vi "Main.vi"() -> ()   [LabVIEW 2018] (continued)
                w3602 = u8 132 items=["I/O (P)"=128, "Input (I)"=129, "Output (Q)"=130, "Bit Memory (M)"=131, "Data (DB)"=132, "Instance Data (DI)"=133, "Local Data (L)"=134, "Predecessor Local Data (VL)"=135] ("寄存器类型")
                w3601 = u16 1 items=["byte", "word", "Dword"] ("数据类型")
                n980 = Index Array(array=w3596) -> (element=w3595:string)  [unwired: 1 in]
                n981 = Decimal String To Number(string=w3595, default (0L)=u32 0 ("默认(0 I32)")) -> (number=w3605:u32)  [unwired: 1 in, 1 out]
                n982 = call "S7_Write.vi"("TCP"=w3597, "寄存器类型"=w3602, "DB #"=u16 20, "写入地址"=u32 2, "数据类型"=w3601, "写入数据"=w3605) -> ("TCP"=w3599:refnum<k5>, "error out"=w3598:errorcluster)  [unwired: 7 in, 1 out]
              }
            }
            "扫码请求回复401" <- w3555
            n983 = Bundle By Name(cluster=w3554, "扫码超时1"=w3555) -> (w3553:T7)
          }
          frame "-------------" {
          }
          frame "读数据保存请求" {
            w3639 = u16 0 items=["byte", "word", "Dword"] ("数据类型")
            w3641 = u8 132 items=["I/O (P)"=128, "Input (I)"=129, "Output (Q)"=130, "Bit Memory (M)"=131, "Data (DB)"=132, "Instance Data (DI)"=133, "Local Data (L)"=134, "Predecessor Local Data (VL)"=135] ("寄存器类型")
            n984 = call "S7_Read.vi"("TCP"=w3631, "DB #"=u16 20, "读取长度"=u16 1, "寄存器类型"=w3641, "起始地址"=u32 0, "数据类型"=w3639) -> ("TCP"=w3630:refnum<k5>, "数据"=w3636:u32[], "error out"=w3629:errorcluster)  [unwired: 6 in, 1 out]
            n985 = Index Array(array=w3636, index=0 ("索引")) -> (element=w3634:u32)
            n986 = Number To Boolean Array(number=w3634) -> (Boolean array=w3633:bool[])
            n987 = Unbundle By Name(w3612) -> ("数据保存超时1"=w3613:string)
            n988 = Index Array(array=w3633, index=1 ("索引")) -> (element=w3618:bool)
            "ST401数据读取" <- w3618
            n989 = Not Equal?(x=w3613, y="999") -> (x != y?=w3615:bool)
            n990 = Not(x=w3615) -> (.not. x?=w3616:bool)
            n991 = call <vilib>:"Boolean Crossing PtByPt.vi"("direction"=enum16{"either", "false-true", "true-false"}."false-true", "input"=w3618) -> ("crossing"=w3622:bool)  [unwired: 1 in]
            n992 = call <vilib>:"Boolean Crossing PtByPt.vi"("direction"=enum16{"either", "false-true", "true-false"}."true-false", "input"=w3618) -> ("crossing"=w3623:bool)  [unwired: 1 in]
            n993 = call "已用时间10"("Reset"=w3616) -> ("Time has Elapsed"=w3617:bool)  [unwired: 11 in, 7 out]
            n994 = Insert Into Array(array=bool[] [] ("数组"), index=0 ("索引"), new element #1=w3622, new element #2=w3623) -> (w3626:bool[])
            n995 = Boolean Array To Number(Boolean array=w3626) -> (number=w3627:u32)
            n996 = case shown="2" w3627 {
              tunnel: [cluster{"Data":string[], "State":T1} {"Data"=[], "State"=enum."读扫码请求3"} ("元素") w3646 w3650] -> w3619
              tunnel: w3611 -> [_ w3647 w3651]
              frame 0, Default {
              }
              frame 1 {
                w3646 = cluster{"Data":string[], "State":T1} {"Data"=[], "State"=enum."读数据"} ("元素")
                n997 = Enqueue Element(queue=w3647, element=w3646, timeout in ms (-1)=10 ("超时毫秒(-1)")) -> ()  [unwired: 1 in, 3 out]
              }
              frame 2 {
                w3650 = cluster{"Data":string[], "State":T1} {"Data"=["999"], "State"=enum."数据保存回复"} ("元素")
                n998 = Enqueue Element(queue=w3651, element=w3650, timeout in ms (-1)=10 ("超时毫秒(-1)")) -> ()  [unwired: 1 in, 3 out]
              }
            }
            n999 = case shown="真" w3617 {
              tunnel: w3611 -> [_ w3643]
              frame False {
              }
              frame True {
                n1000 = Enqueue Element(queue=w3643, element=cluster{"Data":string[], "State":T1} {"Data"=["999"], "State"=enum."数据保存回复"} ("元素"), timeout in ms (-1)=10 ("超时毫秒(-1)")) -> ()  [unwired: 1 in, 3 out]
              }
            }
          }
          frame "读数据" {
            w3657 = u16 0 items=["byte", "word", "Dword"] ("数据类型")
            w3659 = u8 132 items=["I/O (P)"=128, "Input (I)"=129, "Output (Q)"=130, "Bit Memory (M)"=131, "Data (DB)"=132, "Instance Data (DI)"=133, "Local Data (L)"=134, "Predecessor Local Data (VL)"=135] ("寄存器类型")
            w3694 = u16 1 items=["byte", "word", "Dword"] ("数据类型")
            w3690 = u8 132 items=["I/O (P)"=128, "Input (I)"=129, "Output (Q)"=130, "Bit Memory (M)"=131, "Data (DB)"=132, "Instance Data (DI)"=133, "Local Data (L)"=134, "Predecessor Local Data (VL)"=135] ("寄存器类型")
            n1001 = call "S7_Read.vi"("TCP"=w3656, "DB #"=u16 20, "读取长度"=u16 1, "寄存器类型"=w3659, "起始地址"=u32 0, "数据类型"=w3657) -> ("TCP"=w3655:refnum<k5>, "数据"=w3666:u32[], "error out"=w3654:errorcluster)  [unwired: 6 in, 1 out]
            n1002 = Index Array(array=w3666, index=0 ("索引")) -> (element=w3667:u32)
            n1003 = Number To Boolean Array(number=w3667) -> (Boolean array=w3668:bool[])
            n1004 = Index Array(array=w3668, index=7 ("索引")) -> (element=w3665:bool)
            n1005 = Equal?(x=w3665, y=TRUE) -> (x = y?=w3653:bool)
            n1006 = case shown="真" w3653 {
              tunnel: [" " "Y"] -> w3652
              frame False {
              }
              frame True {
              }
            }
            n1007 = call "S7_Read.vi"("TCP"=w3655, "DB #"=u16 20, "读取长度"=u16 1, "寄存器类型"=w3690, "起始地址"=u32 6, "数据类型"=w3694, "error in"=w3654) -> ("TCP"=w3676:refnum<k5>, "数据"=w3689:u32[], "error out"=w3679:errorcluster)  [unwired: 5 in, 1 out]
            n1008 = Index Array(array=w3689) -> (element=w3678:u32)  [unwired: 1 in]
            n1009 = Equal?(x=w3678, y=u32 1) -> (x = y?=w3687:bool)
            n1010 = case shown="假" w3687 {
              tunnel: ["NG" "OK"] -> w3677
              frame False {
              }
              frame True {
              }
            }
            n1011 = Format Date/Time String(time format string (%c)="%Y-%m-%d" ("时间格式字符串(%c)")) -> (date/time string=w3681:string)  [unwired: 2 in]
            n1012 = Get Date/Time String() -> (time string=w3680:string)  [unwired: 3 in, 1 out]
            n1013 = Insert Into Array(array=string[] [] ("数组"), index=0 ("索引"), new element #1="401" ("新元素/子数组"), new element #2=w3677, new element #3=w3681, new element #4=w3680, new element #5=w3677, new element #6=w3652) -> (w3686:string[])
            n1014 = Enqueue Element(queue=w3675, element=w3686, error in (no error)=w3679) -> (error out=w3671:errorcluster)  [unwired: 1 in, 2 out]
            n1015 = property on="ST401数据读取（事件）" class="Bool (严格)"(error in=w3671, "Val(Sgnl)"=TRUE ("值(信号)")) -> (error out=w3670:errorcluster)  [unwired: 1 in, 1 out]
          }
          frame "数据保存回复" {
            w3712 = u8 132 items=["I/O (P)"=128, "Input (I)"=129, "Output (Q)"=130, "Bit Memory (M)"=131, "Data (DB)"=132, "Instance Data (DI)"=133, "Local Data (L)"=134, "Predecessor Local Data (VL)"=135] ("寄存器类型")
            w3713 = u16 1 items=["byte", "word", "Dword"] ("数据类型")
            n1016 = Index Array(array=w3706, index=0 ("索引")) -> (element=w3699:string)
            "数据保存请求回复401" <- w3699
            n1017 = Decimal String To Number(string=w3699, default (0L)=u32 0 ("默认(0 I32)")) -> (number=w3708:u32)  [unwired: 1 in, 1 out]
            n1018 = call "S7_Write.vi"("TCP"=w3707, "寄存器类型"=w3712, "DB #"=u16 20, "写入地址"=u32 4, "数据类型"=w3713, "写入数据"=w3708) -> ("TCP"=w3704:refnum<k5>, "error out"=w3705:errorcluster)  [unwired: 7 in, 1 out]
            n1019 = Bundle By Name(cluster=w3701, "数据保存超时1"=w3699) -> (w3700:T7)
          }
          frame "-----------------" {
          }
          frame "错误" {
            n1020 = Flush Queue(queue=w3722) -> ()  [unwired: 1 in, 3 out]
            n1021 = Flush Queue(queue=w3721) -> ()  [unwired: 1 in, 3 out]
            n1022 = call "S7_Close.vi"("TCP Connection Ref"=w3725) -> ("error out"=w3723:errorcluster)  [unwired: 10 in]
            n1023 = call <vilib>:"Clear Errors.vi"("error in (no error)"=w3723) -> ()  [unwired: 5 in, 2 out]
          }
          frame "退出" {
            n1024 = Release Queue(queue=w3734) -> ()  [unwired: 2 in, 3 out]
            n1025 = Release Queue(queue=w3733) -> ()  [unwired: 2 in, 3 out]
            n1026 = call "S7_Close.vi"("TCP Connection Ref"=w3732) -> ("error out"=w3731:errorcluster)  [unwired: 10 in]
          }
          frame "-------------------" {
          }
          frame "读扫码请求2" {
            w3770 = u16 0 items=["byte", "word", "Dword"] ("数据类型")
            w3772 = u8 132 items=["I/O (P)"=128, "Input (I)"=129, "Output (Q)"=130, "Bit Memory (M)"=131, "Data (DB)"=132, "Instance Data (DI)"=133, "Local Data (L)"=134, "Predecessor Local Data (VL)"=135] ("寄存器类型")
            n1027 = call "S7_Read.vi"("TCP"=w3753, "DB #"=u16 20, "读取长度"=u16 1, "寄存器类型"=w3772, "起始地址"=u32 0, "数据类型"=w3770) -> ("TCP"=w3752:refnum<k5>, "数据"=w3767:u32[], "error out"=w3751:errorcluster)  [unwired: 6 in, 1 out]
            n1028 = Index Array(array=w3767, index=0 ("索引")) -> (element=w3765:u32)
            n1029 = Number To Boolean Array(number=w3765) -> (Boolean array=w3764:bool[])
            n1030 = Index Array(array=w3764, index=2 ("索引")) -> (element=w3754:bool)
            "ST402扫码请求" <- w3754
            n1031 = Unbundle By Name(w3743) -> ("扫码超时2"=w3744:string)
            n1032 = Not Equal?(x=w3744, y="999") -> (x != y?=w3746:bool)
            n1033 = Not(x=w3746) -> (.not. x?=w3747:bool)
            n1034 = call <vilib>:"Boolean Crossing PtByPt.vi"("direction"=enum16{"either", "false-true", "true-false"}."false-true", "input"=w3754) -> ("crossing"=w3760:bool)  [unwired: 1 in]
            n1035 = call <vilib>:"Boolean Crossing PtByPt.vi"("direction"=enum16{"either", "false-true", "true-false"}."true-false", "input"=w3754) -> ("crossing"=w3759:bool)  [unwired: 1 in]
            n1036 = call "已用时间25"("Reset"=w3747) -> ("Time has Elapsed"=w3748:bool)  [unwired: 11 in, 7 out]
            n1037 = Insert Into Array(array=bool[] [] ("数组"), index=0 ("索引"), new element #1=w3760, new element #2=w3759) -> (w3756:bool[])
            n1038 = Boolean Array To Number(Boolean array=w3756) -> (number=w3755:u32)
            n1039 = case shown="0, 默认" w3755 {
              tunnel: [cluster{"Data":string[], "State":T1} {"Data"=[], "State"=enum."读数据保存请求2"} ("元素") w3778 w3780] -> w3750
              tunnel: w3742 -> [_ w3779 w3781]
              frame 0, Default {
              }
              frame 1 {
                w3778 = cluster{"Data":string[], "State":T1} {"Data"=[], "State"=enum."读二维码2"} ("元素")
                n1040 = Enqueue Element(queue=w3779, element=w3778, timeout in ms (-1)=10 ("超时毫秒(-1)")) -> ()  [unwired: 1 in, 3 out]
              }
              frame 2 {
                w3780 = cluster{"Data":string[], "State":T1} {"Data"=["999"], "State"=enum."扫码回复2"} ("元素")
                n1041 = Enqueue Element(queue=w3781, element=w3780, timeout in ms (-1)=10 ("超时毫秒(-1)")) -> ()  [unwired: 1 in, 3 out]
              }
            }
            n1042 = case shown="真" w3748 {
              tunnel: w3742 -> [_ w3774]
              frame False {
              }
              frame True {
                n1043 = Enqueue Element(queue=w3774, element=cluster{"Data":string[], "State":T1} {"Data"=["999"], "State"=enum."扫码回复2"} ("元素"), timeout in ms (-1)=10 ("超时毫秒(-1)")) -> ()  [unwired: 1 in, 3 out]
              }
            }
          }
          frame "读二维码2" {
            n1044 = disable-structure shown="禁用" {
              disable-tunnel: w3791 -> [w3798 _]
              disable-tunnel: w3790 -> [w3797 _]
              disable-tunnel: [w3796 _] -> w3789
              disable-tunnel: [w3795 _] -> w3785
              frame Disabled {
                w3807 = u16 0 items=["byte", "word", "Dword"] ("数据类型")
                w3803 = u8 132 items=["I/O (P)"=128, "Input (I)"=129, "Output (Q)"=130, "Bit Memory (M)"=131, "Data (DB)"=132, "Instance Data (DI)"=133, "Local Data (L)"=134, "Predecessor Local Data (VL)"=135] ("寄存器类型")
                n1045 = call "S7_Read.vi"("TCP"=w3797, "DB #"=u16 20, "读取长度"=u16 17, "寄存器类型"=w3803, "起始地址"=u32 42, "数据类型"=w3807) -> ("TCP"=w3796:refnum<k5>, "数据"=w3808:u32[], "error out"=w3810:errorcluster)  [unwired: 6 in, 1 out]
                n1046 = To Unsigned Word Integer(number=w3808) -> (unsigned 16bit integer=w3809:u16[])
                n1047 = call "还原为字符串.vi"("error in (no error)"=w3810, "输入数组"=w3809) -> ("error out"=w3799:errorcluster, "字符串"=w3793:string)  [unwired: 8 in]
                n1048 = Match Pattern(string=w3793, regular expression=" " ("正则表达式")) -> (before substring=w3792:string)  [unwired: 1 in, 3 out]
                "402二维码 2" <- w3792
                n1049 = Insert Into Array(array=string[] [] ("数组"), index=0 ("索引"), new element=w3792) -> (w3800:string[])
                n1050 = Enqueue Element(queue=w3798, element=w3800, error in (no error)=w3799) -> (error out=w3795:errorcluster)  [unwired: 1 in, 2 out]
              }
              frame Enabled {
              }
            }
            n1051 = property on="ST402扫码请求(事件)" class="Bool (严格)"(error in=w3785, "Val(Sgnl)"=TRUE ("值(信号)")) -> (error out=w3784:errorcluster)  [unwired: 1 in, 1 out]
          }
          frame "扫码回复2" {
            n1052 = Array Size(array=w3819) -> (size(s)=w3820:i32)
            n1053 = case shown="3, 默认" w3820 {
              tunnel: w3819 -> [w3845 w3854]
              tunnel: w3818 -> [w3832 w3855]
              tunnel: [w3823 w3857] -> w3817
              tunnel: [w3822 w3856] -> w3816
              tunnel: [w3821 w3853] -> w3811
              frame 3, Default {
                w3835 = u8 132 items=["I/O (P)"=128, "Input (I)"=129, "Output (Q)"=130, "Bit Memory (M)"=131, "Data (DB)"=132, "Instance Data (DI)"=133, "Local Data (L)"=134, "Predecessor Local Data (VL)"=135] ("寄存器类型")
                w3834 = u16 1 items=["byte", "word", "Dword"] ("数据类型")
                w3842 = u8 132 items=["I/O (P)"=128, "Input (I)"=129, "Output (Q)"=130, "Bit Memory (M)"=131, "Data (DB)"=132, "Instance Data (DI)"=133, "Local Data (L)"=134, "Predecessor Local Data (VL)"=135] ("寄存器类型")
                w3843 = u16 1 items=["byte", "word", "Dword"] ("数据类型")
                w3849 = u8 132 items=["I/O (P)"=128, "Input (I)"=129, "Output (Q)"=130, "Bit Memory (M)"=131, "Data (DB)"=132, "Instance Data (DI)"=133, "Local Data (L)"=134, "Predecessor Local Data (VL)"=135] ("寄存器类型")
                w3848 = u16 1 items=["byte", "word", "Dword"] ("数据类型")
                n1054 = Index Array(array=w3845) -> (element #1=w3821:string, element #2=w3828:string, element #3=w3827:string)  [unwired: 3 in]
                n1055 = Equal?(x=w3827, y="OK") -> (x = y?=w3825:bool)
                n1056 = Decimal String To Number(string=w3828, default (0L)=u32 0 ("默认(0 I32)")) -> (number=w3829:u32)  [unwired: 1 in, 1 out]
                n1057 = case shown="假" w3825 {
                  tunnel: [u32 2 ("写入数据") u32 1 ("写入数据")] -> w3824
                  frame False {
                  }
                  frame True {
                  }
                }
                n1058 = call "S7_Write.vi"("TCP"=w3832, "寄存器类型"=w3849, "DB #"=u16 20, "写入地址"=u32 18, "数据类型"=w3848, "写入数据"=w3829) -> ("TCP"=w3839:refnum<k5>, "error out"=w3840:errorcluster)  [unwired: 7 in, 1 out]
                n1059 = call "S7_Write.vi"("TCP"=w3839, "寄存器类型"=w3842, "DB #"=u16 20, "写入地址"=u32 20, "数据类型"=w3843, "写入数据"=w3824, "error in"=w3840) -> ("TCP"=w3831:refnum<k5>, "error out"=w3830:errorcluster)  [unwired: 6 in, 1 out]
                n1060 = Decimal String To Number(string=w3821, default (0L)=u32 0 ("默认(0 I32)")) -> (number=w3838:u32)  [unwired: 1 in, 1 out]
                n1061 = call "S7_Write.vi"("TCP"=w3831, "寄存器类型"=w3835, "DB #"=u16 20, "写入地址"=u32 14, "数据类型"=w3834, "写入数据"=w3838, "error in"=w3830) -> ("TCP"=w3823:refnum<k5>, "error out"=w3822:errorcluster)  [unwired: 6 in, 1 out]
              }
              frame 1 {
                w3860 = u8 132 items=["I/O (P)"=128, "Input (I)"=129, "Output (Q)"=130, "Bit Memory (M)"=131, "Data (DB)"=132, "Instance Data (DI)"=133, "Local Data (L)"=134, "Predecessor Local Data (VL)"=135] ("寄存器类型")
                w3859 = u16 1 items=["byte", "word", "Dword"] ("数据类型")
                n1062 = Index Array(array=w3854) -> (element=w3853:string)  [unwired: 1 in]
                n1063 = Decimal String To Number(string=w3853, default (0L)=u32 0 ("默认(0 I32)")) -> (number=w3863:u32)  [unwired: 1 in, 1 out]
                n1064 = call "S7_Write.vi"("TCP"=w3855, "寄存器类型"=w3860, "DB #"=u16 20, "写入地址"=u32 14, "数据类型"=w3859, "写入数据"=w3863) -> ("TCP"=w3857:refnum<k5>, "error out"=w3856:errorcluster)  [unwired: 7 in, 1 out]
              }
            }
            "扫码请求回复402" <- w3811
            n1065 = Bundle By Name(cluster=w3813, "扫码超时2"=w3811) -> (w3812:T7)
          }
          frame "-- --------------" {
          }
          frame "读数据保存请求2" {
            w3882 = u8 132 items=["I/O (P)"=128, "Input (I)"=129, "Output (Q)"=130, "Bit Memory (M)"=131, "Data (DB)"=132, "Instance Data (DI)"=133, "Local Data (L)"=134, "Predecessor Local Data (VL)"=135] ("寄存器类型")
            w3881 = u16 1 items=["byte", "word", "Dword"] ("数据类型")
            w3910 = u16 0 items=["byte", "word", "Dword"] ("数据类型")
            w3912 = u8 132 items=["I/O (P)"=128, "Input (I)"=129, "Output (Q)"=130, "Bit Memory (M)"=131, "Data (DB)"=132, "Instance Data (DI)"=133, "Local Data (L)"=134, "Predecessor Local Data (VL)"=135] ("寄存器类型")
            n1066 = Unbundle By Name(w3871) -> ("看门狗"=w3879:string)
            n1067 = Decimal String To Number(string=w3879) -> (number=w3878:i32)  [unwired: 2 in, 1 out]
            n1068 = Equal?(x=w3878, y=0) -> (x = y?=w3876:bool)
            n1069 = case shown="假" w3876 {
              tunnel: [0 ("y") 1 ("y")] -> w3869
              frame False {
              }
              frame True {
              }
            }
            n1070 = call "S7_Write.vi"("TCP"=w3874, "寄存器类型"=w3882, "DB #"=u16 20, "写入地址"=u32 22, "数据类型"=w3881, "写入数据"=w3869) -> ("TCP"=w3873:refnum<k5>, "error out"=w3872:errorcluster)  [unwired: 7 in, 1 out]
            n1071 = local write "40"(w3869) -> ()
            n1072 = Number To Decimal String(number=w3869) -> (decimal integer string=w3875:string)  [unwired: 1 in]
            n1073 = Bundle By Name(cluster=w3871, "看门狗"=w3875) -> (w3870:T7)
            n1074 = call "S7_Read.vi"("TCP"=w3873, "DB #"=u16 20, "读取长度"=u16 1, "寄存器类型"=w3912, "起始地址"=u32 0, "数据类型"=w3910, "error in"=w3872) -> ("TCP"=w3893:refnum<k5>, "数据"=w3907:u32[], "error out"=w3892:errorcluster)  [unwired: 5 in, 1 out]
            n1075 = Index Array(array=w3907, index=0 ("索引")) -> (element=w3905:u32)
            n1076 = Number To Boolean Array(number=w3905) -> (Boolean array=w3904:bool[])
            n1077 = Unbundle By Name(w3870) -> ("数据保存超时2"=w3885:string)
            n1078 = Index Array(array=w3904, index=3 ("索引")) -> (element=w3894:bool)
            "ST402数据读取" <- w3894
            n1079 = Not Equal?(x=w3885, y="999") -> (x != y?=w3887:bool)
            n1080 = Not(x=w3887) -> (.not. x?=w3888:bool)
            n1081 = call <vilib>:"Boolean Crossing PtByPt.vi"("direction"=enum16{"either", "false-true", "true-false"}."false-true", "input"=w3894) -> ("crossing"=w3897:bool)  [unwired: 1 in]
            n1082 = call <vilib>:"Boolean Crossing PtByPt.vi"("direction"=enum16{"either", "false-true", "true-false"}."true-false", "input"=w3894) -> ("crossing"=w3898:bool)  [unwired: 1 in]
            n1083 = call "已用时间26"("Reset"=w3888) -> ("Time has Elapsed"=w3889:bool)  [unwired: 11 in, 7 out]
            n1084 = Insert Into Array(array=bool[] [] ("数组"), index=0 ("索引"), new element #1=w3897, new element #2=w3898) -> (w3901:bool[])
            n1085 = Boolean Array To Number(Boolean array=w3901) -> (number=w3902:u32)
            n1086 = case shown="1" w3902 {
              tunnel: [cluster{"Data":string[], "State":T1} {"Data"=[], "State"=enum."读扫码请求3"} ("元素") w3920 w3923] -> w3891
              tunnel: w3884 -> [_ w3921 w3924]
              frame 0, Default {
              }
              frame 1 {
                w3920 = cluster{"Data":string[], "State":T1} {"Data"=[], "State"=enum."读数据2"} ("元素")
                n1087 = Enqueue Element(queue=w3921, element=w3920, timeout in ms (-1)=10 ("超时毫秒(-1)")) -> ()  [unwired: 1 in, 3 out]
              }
              frame 2 {
                w3923 = cluster{"Data":string[], "State":T1} {"Data"=["999"], "State"=enum."数据保存回复2"} ("元素")
                n1088 = Enqueue Element(queue=w3924, element=w3923, timeout in ms (-1)=10 ("超时毫秒(-1)")) -> ()  [unwired: 1 in, 3 out]
              }
            }
            n1089 = case shown="真" w3889 {
              tunnel: w3884 -> [_ w3916]
              frame False {
              }
              frame True {
                n1090 = Enqueue Element(queue=w3916, element=cluster{"Data":string[], "State":T1} {"Data"=["999"], "State"=enum."数据保存回复2"} ("元素"), timeout in ms (-1)=10 ("超时毫秒(-1)")) -> ()  [unwired: 1 in, 3 out]
              }
            }
          }
          frame "读数据2" {
            n1091 = disable-structure shown="禁用" {
              disable-tunnel: w3931 -> [w3952 _]
              disable-tunnel: [w3937 _] -> w3929
              disable-tunnel: w3928 -> [w3935 _]
              disable-tunnel: [w3934 _] -> w3927
              frame Disabled {
                w3941 = u16 1 items=["byte", "word", "Dword"] ("数据类型")
                w3945 = u8 132 items=["I/O (P)"=128, "Input (I)"=129, "Output (Q)"=130, "Bit Memory (M)"=131, "Data (DB)"=132, "Instance Data (DI)"=133, "Local Data (L)"=134, "Predecessor Local Data (VL)"=135] ("寄存器类型")
                n1092 = call "S7_Read.vi"("TCP"=w3935, "DB #"=u16 20, "读取长度"=u16 1, "寄存器类型"=w3945, "起始地址"=u32 12, "数据类型"=w3941) -> ("TCP"=w3937:refnum<k5>, "数据"=w3940:u32[], "error out"=w3936:errorcluster)  [unwired: 6 in, 1 out]
                n1093 = Index Array(array=w3940) -> (element=w3939:u32)  [unwired: 1 in]
                n1094 = Equal?(x=w3939, y=u32 1) -> (x = y?=w3954:bool)
                n1095 = case shown="真" w3954 {
                  tunnel: ["NG" "OK"] -> w3938
                  frame False {
                  }
                  frame True {
                  }
                }
                n1096 = Format Date/Time String(time format string (%c)="%Y-%m-%d" ("时间格式字符串(%c)")) -> (date/time string=w3947:string)  [unwired: 2 in]
                n1097 = Get Date/Time String() -> (time string=w3946:string)  [unwired: 3 in, 1 out]
                n1098 = Insert Into Array(array=string[] [] ("数组"), index=0 ("索引"), new element #1="402" ("新元素/子数组"), new element #2=w3938, new element #3=w3947, new element #4=w3946, new element #5=w3938) -> (w3953:string[])
                n1099 = Enqueue Element(queue=w3952, element=w3953, error in (no error)=w3936) -> (error out=w3934:errorcluster)  [unwired: 1 in, 2 out]
              }
              frame Enabled {
              }
            }
            n1100 = property on="ST402数据读取（事件）" class="Bool (严格)"(error in=w3927, "Val(Sgnl)"=TRUE ("值(信号)")) -> (error out=w3926:errorcluster)  [unwired: 1 in, 1 out]
          }
          frame "数据保存回复2" {
            w3971 = u8 132 items=["I/O (P)"=128, "Input (I)"=129, "Output (Q)"=130, "Bit Memory (M)"=131, "Data (DB)"=132, "Instance Data (DI)"=133, "Local Data (L)"=134, "Predecessor Local Data (VL)"=135] ("寄存器类型")
            w3972 = u16 1 items=["byte", "word", "Dword"] ("数据类型")
            n1101 = Index Array(array=w3965, index=0 ("索引")) -> (element=w3958:string)
            "数据保存请求回复402" <- w3958
            n1102 = Decimal String To Number(string=w3958, default (0L)=u32 0 ("默认(0 I32)")) -> (number=w3967:u32)  [unwired: 1 in, 1 out]
            n1103 = Bundle By Name(cluster=w3960, "数据保存超时2"=w3958) -> (w3959:T7)
            n1104 = call "S7_Write.vi"("TCP"=w3966, "寄存器类型"=w3971, "DB #"=u16 20, "写入地址"=u32 16, "数据类型"=w3972, "写入数据"=w3967) -> ("TCP"=w3964:refnum<k5>, "error out"=w3963:errorcluster)  [unwired: 7 in, 1 out]
          }
          frame "------------" {
          }
          frame "读扫码请求3" {
            w4007 = u16 0 items=["byte", "word", "Dword"] ("数据类型")
            w4009 = u8 132 items=["I/O (P)"=128, "Input (I)"=129, "Output (Q)"=130, "Bit Memory (M)"=131, "Data (DB)"=132, "Instance Data (DI)"=133, "Local Data (L)"=134, "Predecessor Local Data (VL)"=135] ("寄存器类型")
            n1105 = call "S7_Read.vi"("TCP"=w3990, "DB #"=u16 20, "读取长度"=u16 1, "寄存器类型"=w4009, "起始地址"=u32 0, "数据类型"=w4007) -> ("TCP"=w3989:refnum<k5>, "数据"=w4004:u32[], "error out"=w3988:errorcluster)  [unwired: 6 in, 1 out]
            n1106 = Index Array(array=w4004, index=0 ("索引")) -> (element=w4002:u32)
            n1107 = Number To Boolean Array(number=w4002) -> (Boolean array=w4001:bool[])
            n1108 = Index Array(array=w4001, index=4 ("索引")) -> (element=w3991:bool)
            "ST403扫码请求" <- w3991
            n1109 = Unbundle By Name(w3980) -> ("扫码超时3"=w3981:string)
            n1110 = Not Equal?(x=w3981, y="999") -> (x != y?=w3983:bool)
            n1111 = Not(x=w3983) -> (.not. x?=w3984:bool)
            n1112 = call <vilib>:"Boolean Crossing PtByPt.vi"("direction"=enum16{"either", "false-true", "true-false"}."false-true", "input"=w3991) -> ("crossing"=w3997:bool)  [unwired: 1 in]
            n1113 = call <vilib>:"Boolean Crossing PtByPt.vi"("direction"=enum16{"either", "false-true", "true-false"}."true-false", "input"=w3991) -> ("crossing"=w3996:bool)  [unwired: 1 in]
            n1114 = call "已用时间27"("Reset"=w3984) -> ("Time has Elapsed"=w3985:bool)  [unwired: 11 in, 7 out]
            n1115 = Insert Into Array(array=bool[] [] ("数组"), index=0 ("索引"), new element #1=w3997, new element #2=w3996) -> (w3993:bool[])
            n1116 = Boolean Array To Number(Boolean array=w3993) -> (number=w3992:u32)
            n1117 = case shown="2" w3992 {
              tunnel: [cluster{"Data":string[], "State":T1} {"Data"=[], "State"=enum."读数据保存请求3"} ("元素") w4015 w4017] -> w3987
              tunnel: w3979 -> [_ w4016 w4018]
              frame 0, Default {
              }
              frame 1 {
                w4015 = cluster{"Data":string[], "State":T1} {"Data"=[], "State"=enum."读二维码3"} ("元素")
                n1118 = Enqueue Element(queue=w4016, element=w4015, timeout in ms (-1)=10 ("超时毫秒(-1)")) -> ()  [unwired: 1 in, 3 out]
              }
              frame 2 {
                w4017 = cluster{"Data":string[], "State":T1} {"Data"=["999"], "State"=enum."扫码回复3"} ("元素")
                n1119 = Enqueue Element(queue=w4018, element=w4017, timeout in ms (-1)=10 ("超时毫秒(-1)")) -> ()  [unwired: 1 in, 3 out]
              }
            }
            n1120 = case shown="真" w3985 {
              tunnel: w3979 -> [_ w4011]
              frame False {
              }
              frame True {
                n1121 = Enqueue Element(queue=w4011, element=cluster{"Data":string[], "State":T1} {"Data"=["999"], "State"=enum."扫码回复3"} ("元素"), timeout in ms (-1)=10 ("超时毫秒(-1)")) -> ()  [unwired: 1 in, 3 out]
              }
            }
          }
          frame "读二维码3" {
            w4035 = u16 0 items=["byte", "word", "Dword"] ("数据类型")
            w4031 = u8 132 items=["I/O (P)"=128, "Input (I)"=129, "Output (Q)"=130, "Bit Memory (M)"=131, "Data (DB)"=132, "Instance Data (DI)"=133, "Local Data (L)"=134, "Predecessor Local Data (VL)"=135] ("寄存器类型")
            n1122 = call "S7_Read.vi"("TCP"=w4030, "DB #"=u16 20, "读取长度"=u16 17, "寄存器类型"=w4031, "起始地址"=u32 60, "数据类型"=w4035) -> ("TCP"=w4029:refnum<k5>, "数据"=w4036:u32[], "error out"=w4038:errorcluster)  [unwired: 6 in, 1 out]
            n1123 = To Unsigned Word Integer(number=w4036) -> (unsigned 16bit integer=w4037:u16[])
            n1124 = call "还原为字符串.vi"("error in (no error)"=w4038, "输入数组"=w4037) -> ("error out"=w4022:errorcluster, "字符串"=w4023:string)  [unwired: 8 in]
            n1125 = Match Pattern(string=w4023, regular expression=" " ("正则表达式")) -> (before substring=w4020:string)  [unwired: 1 in, 3 out]
            n1126 = flat-sequence {
              tunnel: w4022 -> [w4040]
              tunnel: [w4040] -> w4021
              tunnel: w4020 -> [w4039]
              tunnel: [w4043] -> w4025
              tunnel: w4021 -> [w4041]
              frame #0 {
                "403二维码" <- w4039
              }
              frame #1 {
                n1127 = property on="ST403扫码请求(事件)" class="Bool (严格)"(error in=w4041, "Val(Sgnl)"=TRUE ("值(信号)")) -> (error out=w4043:errorcluster)  [unwired: 1 in, 1 out]
              }
            }
          }
          frame "扫码回复3" {
            n1128 = Array Size(array=w4046) -> (size(s)=w4053:i32)
            n1129 = case shown="3, 默认" w4053 {
              tunnel: w4046 -> [w4078 w4087]
              tunnel: w4050 -> [w4065 w4088]
              tunnel: [w4056 w4090] -> w4048
              tunnel: [w4055 w4089] -> w4047
              tunnel: [w4054 w4086] -> w4052
              frame 3, Default {
                w4068 = u8 132 items=["I/O (P)"=128, "Input (I)"=129, "Output (Q)"=130, "Bit Memory (M)"=131, "Data (DB)"=132, "Instance Data (DI)"=133, "Local Data (L)"=134, "Predecessor Local Data (VL)"=135] ("寄存器类型")
                w4067 = u16 1 items=["byte", "word", "Dword"] ("数据类型")
                w4075 = u8 132 items=["I/O (P)"=128, "Input (I)"=129, "Output (Q)"=130, "Bit Memory (M)"=131, "Data (DB)"=132, "Instance Data (DI)"=133, "Local Data (L)"=134, "Predecessor Local Data (VL)"=135] ("寄存器类型")
                w4076 = u16 1 items=["byte", "word", "Dword"] ("数据类型")
                w4082 = u8 132 items=["I/O (P)"=128, "Input (I)"=129, "Output (Q)"=130, "Bit Memory (M)"=131, "Data (DB)"=132, "Instance Data (DI)"=133, "Local Data (L)"=134, "Predecessor Local Data (VL)"=135] ("寄存器类型")
                w4081 = u16 1 items=["byte", "word", "Dword"] ("数据类型")
                n1130 = Index Array(array=w4078) -> (element #1=w4054:string, element #2=w4061:string, element #3=w4060:string)  [unwired: 3 in]
                n1131 = Equal?(x=w4060, y="OK") -> (x = y?=w4058:bool)
                n1132 = Decimal String To Number(string=w4061, default (0L)=u32 0 ("默认(0 I32)")) -> (number=w4062:u32)  [unwired: 1 in, 1 out]
                n1133 = case shown="假" w4058 {
                  tunnel: [u32 2 ("写入数据") u32 1 ("写入数据")] -> w4057
                  frame False {
                  }
                  frame True {
                  }
                }
                n1134 = call "S7_Write.vi"("TCP"=w4065, "寄存器类型"=w4082, "DB #"=u16 20, "写入地址"=u32 84, "数据类型"=w4081, "写入数据"=w4062) -> ("TCP"=w4072:refnum<k5>, "error out"=w4073:errorcluster)  [unwired: 7 in, 1 out]
                n1135 = call "S7_Write.vi"("TCP"=w4072, "寄存器类型"=w4075, "DB #"=u16 20, "写入地址"=u32 86, "数据类型"=w4076, "写入数据"=w4057, "error in"=w4073) -> ("TCP"=w4064:refnum<k5>, "error out"=w4063:errorcluster)  [unwired: 6 in, 1 out]
                n1136 = Decimal String To Number(string=w4054, default (0L)=u32 0 ("默认(0 I32)")) -> (number=w4071:u32)  [unwired: 1 in, 1 out]
                n1137 = call "S7_Write.vi"("TCP"=w4064, "寄存器类型"=w4068, "DB #"=u16 20, "写入地址"=u32 78, "数据类型"=w4067, "写入数据"=w4071, "error in"=w4063) -> ("TCP"=w4056:refnum<k5>, "error out"=w4055:errorcluster)  [unwired: 6 in, 1 out]
              }
              frame 1 {
                w4093 = u8 132 items=["I/O (P)"=128, "Input (I)"=129, "Output (Q)"=130, "Bit Memory (M)"=131, "Data (DB)"=132, "Instance Data (DI)"=133, "Local Data (L)"=134, "Predecessor Local Data (VL)"=135] ("寄存器类型")
                w4092 = u16 1 items=["byte", "word", "Dword"] ("数据类型")
                n1138 = Index Array(array=w4087) -> (element=w4086:string)  [unwired: 1 in]
                n1139 = Decimal String To Number(string=w4086, default (0L)=u32 0 ("默认(0 I32)")) -> (number=w4096:u32)  [unwired: 1 in, 1 out]
                n1140 = call "S7_Write.vi"("TCP"=w4088, "寄存器类型"=w4093, "DB #"=u16 20, "写入地址"=u32 78, "数据类型"=w4092, "写入数据"=w4096) -> ("TCP"=w4090:refnum<k5>, "error out"=w4089:errorcluster)  [unwired: 7 in, 1 out]
              }
            }
            "扫码请求回复403" <- w4052
            n1141 = Bundle By Name(cluster=w4051, "扫码超时3"=w4052) -> (w4049:T7)
          }
          frame "- ---------" {
          }
          frame "读数据保存请求3" {
            w4130 = u16 0 items=["byte", "word", "Dword"] ("数据类型")
            w4132 = u8 132 items=["I/O (P)"=128, "Input (I)"=129, "Output (Q)"=130, "Bit Memory (M)"=131, "Data (DB)"=132, "Instance Data (DI)"=133, "Local Data (L)"=134, "Predecessor Local Data (VL)"=135] ("寄存器类型")
            n1142 = call "S7_Read.vi"("TCP"=w4108, "DB #"=u16 20, "读取长度"=u16 1, "寄存器类型"=w4132, "起始地址"=u32 0, "数据类型"=w4130) -> ("TCP"=w4104:refnum<k5>, "数据"=w4127:u32[], "error out"=w4106:errorcluster)  [unwired: 6 in, 1 out]
            n1143 = Index Array(array=w4127, index=0 ("索引")) -> (element=w4125:u32)
            n1144 = Number To Boolean Array(number=w4125) -> (Boolean array=w4124:bool[])
            n1145 = Unbundle By Name(w4103) -> ("数据保存超时3"=w4109:string)
            n1146 = Index Array(array=w4124, index=5 ("索引")) -> (element=w4114:bool)
            "ST403数据读取" <- w4114
            n1147 = Not Equal?(x=w4109, y="999") -> (x != y?=w4111:bool)
            n1148 = Not(x=w4111) -> (.not. x?=w4112:bool)
            n1149 = call <vilib>:"Boolean Crossing PtByPt.vi"("direction"=enum16{"either", "false-true", "true-false"}."false-true", "input"=w4114) -> ("crossing"=w4117:bool)  [unwired: 1 in]
            n1150 = call <vilib>:"Boolean Crossing PtByPt.vi"("direction"=enum16{"either", "false-true", "true-false"}."true-false", "input"=w4114) -> ("crossing"=w4118:bool)  [unwired: 1 in]
            n1151 = call "已用时间28"("Reset"=w4112) -> ("Time has Elapsed"=w4113:bool)  [unwired: 11 in, 7 out]
            n1152 = Insert Into Array(array=bool[] [] ("数组"), index=0 ("索引"), new element #1=w4117, new element #2=w4118) -> (w4121:bool[])
            n1153 = Boolean Array To Number(Boolean array=w4121) -> (number=w4122:u32)
            n1154 = case shown="0, 默认" w4122 {
              tunnel: [cluster{"Data":string[], "State":T1} {"Data"=[], "State"=enum."看门狗"} ("元素") w4138 w4141] -> w4105
              tunnel: w4107 -> [_ w4139 w4142]
              frame 0, Default {
              }
              frame 1 {
                w4138 = cluster{"Data":string[], "State":T1} {"Data"=[], "State"=enum."读数据3"} ("元素")
                n1155 = Enqueue Element(queue=w4139, element=w4138, timeout in ms (-1)=10 ("超时毫秒(-1)")) -> ()  [unwired: 1 in, 3 out]
              }
              frame 2 {
                w4141 = cluster{"Data":string[], "State":T1} {"Data"=["999"], "State"=enum."数据保存回复3"} ("元素")
                n1156 = Enqueue Element(queue=w4142, element=w4141, timeout in ms (-1)=10 ("超时毫秒(-1)")) -> ()  [unwired: 1 in, 3 out]
              }
            }
            n1157 = case shown="真" w4113 {
              tunnel: w4107 -> [_ w4134]
              frame False {
              }
              frame True {
                n1158 = Enqueue Element(queue=w4134, element=cluster{"Data":string[], "State":T1} {"Data"=["999"], "State"=enum."数据保存回复3"} ("元素"), timeout in ms (-1)=10 ("超时毫秒(-1)")) -> ()  [unwired: 1 in, 3 out]
              }
            }
          }
          frame "读数据3" {
            w4162 = u16 0 items=["byte", "word", "Dword"] ("数据类型")
            w4160 = u8 132 items=["I/O (P)"=128, "Input (I)"=129, "Output (Q)"=130, "Bit Memory (M)"=131, "Data (DB)"=132, "Instance Data (DI)"=133, "Local Data (L)"=134, "Predecessor Local Data (VL)"=135] ("寄存器类型")
            w4166 = i16 4 ("精度(6)")
            w4173 = u16 2 items=["byte", "word", "Dword"] ("数据类型")
            w4175 = u8 132 items=["I/O (P)"=128, "Input (I)"=129, "Output (Q)"=130, "Bit Memory (M)"=131, "Data (DB)"=132, "Instance Data (DI)"=133, "Local Data (L)"=134, "Predecessor Local Data (VL)"=135] ("寄存器类型")
            w4199 = u16 1 items=["byte", "word", "Dword"] ("数据类型")
            w4195 = u8 132 items=["I/O (P)"=128, "Input (I)"=129, "Output (Q)"=130, "Bit Memory (M)"=131, "Data (DB)"=132, "Instance Data (DI)"=133, "Local Data (L)"=134, "Predecessor Local Data (VL)"=135] ("寄存器类型")
            n1159 = call "S7_Read.vi"("TCP"=w4157, "DB #"=u16 20, "读取长度"=u16 1, "寄存器类型"=w4160, "起始地址"=u32 0, "数据类型"=w4162) -> ("TCP"=w4156:refnum<k5>, "数据"=w4150:u32[], "error out"=w4155:errorcluster)  [unwired: 6 in, 1 out]
            n1160 = Index Array(array=w4150, index=0 ("索引")) -> (element=w4152:u32)
            n1161 = Number To Boolean Array(number=w4152) -> (Boolean array=w4153:bool[])
            n1162 = Index Array(array=w4153, index=6 ("索引")) -> (element=w4149:bool)
            n1163 = Equal?(x=w4149, y=TRUE) -> (x = y?=w4147:bool)
            n1164 = case shown="假" w4147 {
              tunnel: [" " "Y"] -> w4146
              frame False {
              }
              frame True {
              }
            }
            n1165 = call "S7_Read.vi"("TCP"=w4156, "DB #"=u16 20, "读取长度"=u16 2, "寄存器类型"=w4175, "起始地址"=u32 88, "数据类型"=w4173, "error in"=w4155) -> ("TCP"=w4172:refnum<k5>, "数据"=w4170:u32[], "error out"=w4171:errorcluster)  [unwired: 5 in, 1 out]
            n1166 = Divide(x=w4170, y=u32[] [10000, 10000]) -> (x/y=w4168:dbl[])
            n1167 = Index Array(array=w4168) -> (element #1=w4167:dbl, element #2=w4163:dbl)  [unwired: 2 in]
            n1168 = Number To Fractional String(number=w4167, precision (6)=w4166) -> (F-format string=w4165:string)  [unwired: 2 in]
            n1169 = Number To Fractional String(number=w4163, precision (6)=w4166) -> (F-format string=w4164:string)  [unwired: 2 in]
            n1170 = call "S7_Read.vi"("TCP"=w4172, "DB #"=u16 20, "读取长度"=u16 1, "寄存器类型"=w4195, "起始地址"=u32 82, "数据类型"=w4199, "error in"=w4171) -> ("TCP"=w4182:refnum<k5>, "数据"=w4194:u32[], "error out"=w4145:errorcluster)  [unwired: 5 in, 1 out]
            n1171 = local read "ST40 Circlip 5026621"() -> (w4178:string)
            n1172 = Index Array(array=w4194) -> (element=w4185:u32)  [unwired: 1 in]
            n1173 = Equal?(x=w4185, y=u32 1) -> (x = y?=w4192:bool)
            n1174 = case shown="假" w4192 {
              tunnel: ["NG" "OK"] -> w4184
              frame False {
              }
              frame True {
              }
            }
            n1175 = Format Date/Time String(time format string (%c)="%Y-%m-%d" ("时间格式字符串(%c)")) -> (date/time string=w4187:string)  [unwired: 2 in]
            n1176 = Get Date/Time String() -> (time string=w4186:string)  [unwired: 3 in, 1 out]
            n1177 = Insert Into Array(array=string[] [] ("数组"), index=0 ("索引"), new element #1="403" ("新元素/子数组"), new element #2=w4184, new element #3=w4187, new element #4=w4186, new element #5=w4184, new element #6=w4178, new element #7=w4165, new element #8=w4164, new element #9=w4146) -> (w4143:string[])
            n1178 = flat-sequence {
              tunnel: w4145 -> [w4201]
              tunnel: [w4201] -> w4144
              tunnel: w4143 -> [w4200]
              tunnel: [w4203] -> w4179
              tunnel: w4144 -> [w4202]
              frame #0 {
                "403读取数据" <- w4200
              }
              frame #1 {
                n1179 = property on="ST403数据读取（事件）" class="Bool (严格)"(error in=w4202, "Val(Sgnl)"=TRUE ("值(信号)")) -> (error out=w4203:errorcluster)  [unwired: 1 in, 1 out]
              }
            }
          }
          frame "数据保存回复3" {
            w4222 = u8 132 items=["I/O (P)"=128, "Input (I)"=129, "Output (Q)"=130, "Bit Memory (M)"=131, "Data (DB)"=132, "Instance Data (DI)"=133, "Local Data (L)"=134, "Predecessor Local Data (VL)"=135] ("寄存器类型")
            w4223 = u16 1 items=["byte", "word", "Dword"] ("数据类型")
            n1180 = Index Array(array=w4213, index=0 ("索引")) -> (element=w4217:string)
            "数据保存请求回复403" <- w4217
            n1181 = Decimal String To Number(string=w4217, default (0L)=u32 0 ("默认(0 I32)")) -> (number=w4218:u32)  [unwired: 1 in, 1 out]
            n1182 = call "S7_Write.vi"("TCP"=w4214, "寄存器类型"=w4222, "DB #"=u16 20, "写入地址"=u32 80, "数据类型"=w4223, "写入数据"=w4218) -> ("TCP"=w4212:refnum<k5>, "error out"=w4211:errorcluster)  [unwired: 7 in, 1 out]
            n1183 = Bundle By Name(cluster=w4216, "数据保存超时3"=w4217) -> (w4215:T7)
          }
          frame "----------" {
          }
          frame "看门狗" {
            w4247 = u8 132 items=["I/O (P)"=128, "Input (I)"=129, "Output (Q)"=130, "Bit Memory (M)"=131, "Data (DB)"=132, "Instance Data (DI)"=133, "Local Data (L)"=134, "Predecessor Local Data (VL)"=135] ("寄存器类型")
            w4246 = u16 1 items=["byte", "word", "Dword"] ("数据类型")
            n1184 = Unbundle By Name(w4235) -> ("看门狗"=w4244:string)
            n1185 = Decimal String To Number(string=w4244) -> (number=w4243:i32)  [unwired: 2 in, 1 out]
            n1186 = Equal?(x=w4243, y=0) -> (x = y?=w4241:bool)
            n1187 = case shown="假" w4241 {
              tunnel: [0 ("y") 1 ("y")] -> w4236
              frame False {
              }
              frame True {
              }
            }
            "40" <- w4236
            n1188 = call "S7_Write.vi"("TCP"=w4240, "寄存器类型"=w4247, "DB #"=u16 20, "写入地址"=u32 22, "数据类型"=w4246, "写入数据"=w4236) -> ("TCP"=w4233:refnum<k5>, "error out"=w4231:errorcluster)  [unwired: 7 in, 1 out]
            n1189 = Number To Decimal String(number=w4236) -> (decimal integer string=w4237:string)  [unwired: 1 in]
            n1190 = Bundle By Name(cluster=w4235, "看门狗"=w4237) -> (w4234:T7)
            n1191 = disable-structure shown="启用" {
              disable-tunnel: w4233 -> [w4249 w4253]
              disable-tunnel: [w4249 w4256] -> w4232
              disable-tunnel: w4231 -> [w4250 w4254]
              disable-tunnel: [w4250 w4255] -> w4230
              frame Disabled {
              }
              frame Enabled {
                w4258 = u8 132 items=["I/O (P)"=128, "Input (I)"=129, "Output (Q)"=130, "Bit Memory (M)"=131, "Data (DB)"=132, "Instance Data (DI)"=133, "Local Data (L)"=134, "Predecessor Local Data (VL)"=135] ("寄存器类型")
                w4252 = u16 1 items=["byte", "word", "Dword"] ("数据类型")
                n1192 = local read "80产品型号"() -> (w4251:u32)
                n1193 = call "S7_Write.vi"("TCP"=w4253, "寄存器类型"=w4258, "DB #"=u16 20, "写入地址"=u32 96, "数据类型"=w4252, "写入数据"=w4251, "error in"=w4254) -> ("TCP"=w4256:refnum<k5>, "error out"=w4255:errorcluster)  [unwired: 6 in, 1 out]
              }
            }
          }
        }
      }
      n1194 = while {
        shift-right: [w6506] -> _
        shift-left: cluster{"Data":string[], "State":T1} {"Data"=[], "State"=enum."PLC通讯初始化"} ("元素") -> [w6507]
        shift-right: [w6515] -> _
        shift-left: w143 -> [w6512]
        shift-right: [w6516] -> _
        shift-left: _ -> [w6513]
        tunnel: w141 -> [w6508]
        tunnel: w140 -> [w6503]
        tunnel: w142 -> [_]
        shift-right: [w6502] -> _
        shift-left: _ -> [w6501]
        stop <- w6504 stop-if-true
        # "OP20"
        n1195 = local read "退出"() -> (w6511:bool)
        n1196 = Wait (ms)(milliseconds to wait=u32 20 ("等待时间（毫秒）")) -> ()  [unwired: 1 out]
        n1197 = call "状态判断.vi"("error IO"=w6512, "退出？"=w6511, "簇 输入"=w6507, "队列输入"=w6508) -> ("簇"=w6510:cluster{"Data":string[], "State":T1})  [unwired: 6 in, 1 out]
        n1198 = Unbundle By Name(w6510) -> ("Data"=w6505:string[], "State"=w6509:T1)
        "20 State" <- w6509
        n1199 = case shown="\"PLC通讯初始化\", 默认" w6509 {
          tunnel: [w6524 w6565 w6587 w6618 w6638 w6689 w6709 w6755 w6769 w6783 w6803 w6850 w6870 w6922 w6927 w6985 w7020 w7035 refnum<k5> refnum ("TCP") refnum<k5> refnum ("TCP") w7054] -> w6516
          tunnel: [w6523 errorcluster {"status"=FALSE, "code"=0, "source"=""} ("error out") w6586 w6615 w6637 errorcluster {"status"=FALSE, "code"=0, "source"=""} ("error out") w6708 w6735 w6770 errorcluster {"status"=FALSE, "code"=0, "source"=""} ("error out") w6800 w6849 w6869 errorcluster {"status"=FALSE, "code"=0, "source"=""} ("error out") w6925 w6983 w7019 errorcluster {"status"=FALSE, "code"=0, "source"=""} ("error out") errorcluster {"status"=FALSE, "code"=0, "source"=""} ("error out") w7047 w7055] -> w6515
          tunnel: w6513 -> [_ w6565 w6588 w6619 w6639 w6689 w6710 w6734 w6771 w6783 w6788 w6852 w6873 w6922 w6929 w6986 w7023 w7035 w7042 w7049 w7090]
          tunnel: w6508 -> [w6550 _ w6568 _ _ _ w6690 _ _ _ w6799 _ _ _ w6928 _ _ _ w7038 w7050 _]
          tunnel: [cluster{"Data":string[], "State":T1} {"Data"=[], "State"=enum."读扫码请求"} ("元素") cluster{"Data":string[], "State":T1} {"Data"=[], "State"=enum."读扫码请求"} ("元素") w6576 cluster{"Data":string[], "State":T1} {"Data"=[], "State"=enum."读数据保存请求"} ("元素") cluster{"Data":string[], "State":T1} {"Data"=[], "State"=enum."读数据保存请求"} ("元素") cluster{"Data":string[], "State":T1} {"Data"=[], "State"=enum."读数据保存请求"} ("元素") w6698 cluster{"Data":string[], "State":T1} {"Data"=[], "State"=enum."读扫码请求2"} ("元素") cluster{"Data":string[], "State":T1} {"Data"=[], "State"=enum."读扫码请求2"} ("元素") cluster{"Data":string[], "State":T1} {"Data"=[], "State"=enum."读扫码请求2"} ("元素") w6802 cluster{"Data":string[], "State":T1} {"Data"=[], "State"=enum."读数据保存请求2"} ("元素") cluster{"Data":string[], "State":T1} {"Data"=[], "State"=enum."读数据保存请求2"} ("元素") cluster{"Data":string[], "State":T1} {"Data"=[], "State"=enum."PLC通讯初始化"} ("元素") w6924 cluster{"Data":string[], "State":T1} {"Data"=[], "State"=enum."看门狗"} ("元素") cluster{"Data":string[], "State":T1} {"Data"=[], "State"=enum."看门狗"} ("元素") cluster{"Data":string[], "State":T1} {"Data"=[], "State"=enum."看门狗"} ("元素") cluster{"Data":string[], "State":T1} {"Data"=[], "State"=enum."PLC通讯初始化"} ("元素") cluster{"Data":string[], "State":T1} {"Data"=[], "State"=enum."退出"} ("元素") cluster{"Data":string[], "State":T1} {"Data"=[], "State"=enum."读扫码请求"} ("元素")] -> w6506
          tunnel: w6505 -> [_ _ _ _ w6635 _ _ _ w6766 _ _ _ w6872 _ _ _ w7018 _ _ _ _]
          tunnel: [FALSE FALSE FALSE FALSE FALSE FALSE FALSE FALSE FALSE FALSE FALSE FALSE FALSE FALSE FALSE FALSE FALSE FALSE FALSE TRUE FALSE] -> w6504
          tunnel: w6503 -> [_ _ _ _ _ _ _ w6746 _ _ _ _ _ _ _ _ _ _ w7039 w7051 _]
          tunnel: [T11 {"扫码超时1"="999", "数据保存超时1"="999", "看门狗"="0", "扫码超时2"="999", "数据保存超时2"="999"} w6561 w6569 w6614 w6634 w6685 w6691 w6736 w6763 w6779 w6786 w6851 w6867 w6923 w6930 w6992 w7021 w7036 w7037 w7046 w7084] -> w6502
          tunnel: w6501 -> [_ w6561 w6569 w6614 w6634 w6685 w6691 w6736 w6765 w6779 w6787 w6851 w6868 w6923 w6930 w6992 w7022 w7036 w7037 w7046 w7085]
          frame "PLC通讯初始化", Default {
            w6533 = u16 0 items=["byte", "word", "Dword"] ("数据类型")
            w6527 = u8 132 items=["I/O (P)"=128, "Input (I)"=129, "Output (Q)"=130, "Bit Memory (M)"=131, "Data (DB)"=132, "Instance Data (DI)"=133, "Local Data (L)"=134, "Predecessor Local Data (VL)"=135] ("寄存器类型")
            w6542 = u16 0 items=["byte", "word", "Dword"] ("数据类型")
            w6548 = u8 132 items=["I/O (P)"=128, "Input (I)"=129, "Output (Q)"=130, "Bit Memory (M)"=131, "Data (DB)"=132, "Instance Data (DI)"=133, "Local Data (L)"=134, "Predecessor Local Data (VL)"=135] ("寄存器类型")
            w6559 = u8 0 items=["S7-1200.200.200SMART"=0, "S7-300"=2, "S7-400"=3] ("PLC 系列")
            n1200 = call "S7_Open.vi"("IP 地址"="192.168.0.20", "PLC 系列"=w6559, "超时（MS）"=100) -> ("TCP"=w6541:refnum<k5>, "error out"=w6540:errorcluster)  [unwired: 10 in, 1 out]
            n1201 = Unbundle By Name(w6540) -> ("status"=→"ST20通讯状态":bool)
            n1202 = Enqueue Element(queue=w6550, element=cluster{"Data":string[], "State":T1} {"Data"=["999"], "State"=enum."扫码回复"} ("元素")) -> (queue out=w6555:refnum<queue>, error out=w6554:errorcluster)  [unwired: 2 in, 1 out]
            n1203 = Enqueue Element(queue=w6555, element=cluster{"Data":string[], "State":T1} {"Data"=["999"], "State"=enum."数据保存回复"} ("元素"), error in (no error)=w6554) -> (queue out=w6535:refnum<queue>, error out=w6534:errorcluster)  [unwired: 1 in, 1 out]
            n1204 = call "S7_Read.vi"("TCP"=w6541, "DB #"=u16 20, "读取长度"=u16 17, "寄存器类型"=w6548, "起始地址"=u32 24, "数据类型"=w6542, "error in"=w6540) -> ("TCP"=w6525:refnum<k5>, "数据"=w6544:u32[], "error out"=w6526:errorcluster)  [unwired: 5 in, 1 out]
            n1205 = Enqueue Element(queue=w6535, element=cluster{"Data":string[], "State":T1} {"Data"=["999"], "State"=enum."扫码回复2"} ("元素"), error in (no error)=w6534) -> (queue out=w6538:refnum<queue>, error out=w6539:errorcluster)  [unwired: 1 in, 1 out]
            n1206 = To Unsigned Word Integer(number=w6544) -> (unsigned 16bit integer=w6543:u16[])
            n1207 = call "还原为字符串.vi"("输入数组"=w6543) -> ("字符串"=w6521:string)  [unwired: 9 in, 1 out]
            n1208 = Match Pattern(string=w6521, regular expression=" " ("正则表达式")) -> (before substring=w6520:string)  [unwired: 1 in, 3 out]
            n1209 = Enqueue Element(queue=w6538, element=cluster{"Data":string[], "State":T1} {"Data"=["999"], "State"=enum."数据保存回复2"} ("元素"), error in (no error)=w6539) -> ()  [unwired: 1 in, 3 out]
            n1210 = local write "201二维码"(w6520) -> ()
            n1211 = call "S7_Read.vi"("TCP"=w6525, "DB #"=u16 20, "读取长度"=u16 17, "寄存器类型"=w6527, "起始地址"=u32 42, "数据类型"=w6533, "error in"=w6526) -> ("TCP"=w6524:refnum<k5>, "数据"=w6531:u32[], "error out"=w6523:errorcluster)  [unwired: 5 in, 1 out]
            n1212 = To Unsigned Word Integer(number=w6531) -> (unsigned 16bit integer=w6532:u16[])
            n1213 = call "还原为字符串.vi"("输入数组"=w6532) -> ("字符串"=w6518:string)  [unwired: 9 in, 1 out]
            n1214 = Match Pattern(string=w6518, regular expression=" " ("正则表达式")) -> (before substring=w6517:string)  [unwired: 1 in, 3 out]
            n1215 = local write "202二维码"(w6517) -> ()
          }
          frame "--------------" {
          }
          frame "读扫码请求" {
            w6596 = u16 0 items=["byte", "word", "Dword"] ("数据类型")
            w6598 = u8 132 items=["I/O (P)"=128, "Input (I)"=129, "Output (Q)"=130, "Bit Memory (M)"=131, "Data (DB)"=132, "Instance Data (DI)"=133, "Local Data (L)"=134, "Predecessor Local Data (VL)"=135] ("寄存器类型")
            n1216 = call "S7_Read.vi"("TCP"=w6588, "DB #"=u16 20, "读取长度"=u16 1, "寄存器类型"=w6598, "起始地址"=u32 0, "数据类型"=w6596) -> ("TCP"=w6587:refnum<k5>, "数据"=w6593:u32[], "读取成功"=w6566:bool, "error out"=w6586:errorcluster)  [unwired: 6 in]
            n1217 = Not(x=w6566) -> (.not. x?=w6567:bool)
            n1218 = Index Array(array=w6593, index=0 ("索引")) -> (element=w6591:u32)
            n1219 = local write "ST20通讯状态"(w6567) -> ()
            n1220 = Number To Boolean Array(number=w6591) -> (Boolean array=w6590:bool[])
            n1221 = Unbundle By Name(w6569) -> ("扫码超时1"=w6570:string)
            n1222 = Index Array(array=w6590, index=0 ("索引")) -> (element=w6575:bool)
            "ST202扫码请求" <- w6575
            n1223 = Not Equal?(x=w6570, y="999") -> (x != y?=w6572:bool)
            n1224 = Not(x=w6572) -> (.not. x?=w6573:bool)
            n1225 = call <vilib>:"Boolean Crossing PtByPt.vi"("direction"=enum16{"either", "false-true", "true-false"}."false-true", "input"=w6575) -> ("crossing"=w6582:bool)  [unwired: 1 in]
            n1226 = call <vilib>:"Boolean Crossing PtByPt.vi"("direction"=enum16{"either", "false-true", "true-false"}."true-false", "input"=w6575) -> ("crossing"=w6581:bool)  [unwired: 1 in]
            n1227 = call "已用时间5"("Reset"=w6573) -> ("Time has Elapsed"=w6574:bool)  [unwired: 11 in, 7 out]
            n1228 = Insert Into Array(array=bool[] [] ("数组"), index=0 ("索引"), new element #1=w6582, new element #2=w6581) -> (w6578:bool[])
            n1229 = Boolean Array To Number(Boolean array=w6578) -> (number=w6577:u32)
            n1230 = case shown="2" w6577 {
              tunnel: [cluster{"Data":string[], "State":T1} {"Data"=[], "State"=enum."读数据保存请求"} ("元素") w6604 w6606] -> w6576
              tunnel: w6568 -> [_ w6605 w6607]
              frame 0, Default {
              }
              frame 1 {
                w6604 = cluster{"Data":string[], "State":T1} {"Data"=[], "State"=enum."读二维码"} ("元素")
                n1231 = Enqueue Element(queue=w6605, element=w6604, timeout in ms (-1)=10 ("超时毫秒(-1)")) -> ()  [unwired: 1 in, 3 out]
              }
              frame 2 {
                w6606 = cluster{"Data":string[], "State":T1} {"Data"=["999"], "State"=enum."扫码回复"} ("元素")
                n1232 = Enqueue Element(queue=w6607, element=w6606, timeout in ms (-1)=10 ("超时毫秒(-1)")) -> ()  [unwired: 1 in, 3 out]
              }
            }
            n1233 = case shown="真" w6574 {
              tunnel: w6568 -> [_ w6600]
              frame False {
              }
              frame True {
                n1234 = Enqueue Element(queue=w6600, element=cluster{"Data":string[], "State":T1} {"Data"=["999"], "State"=enum."扫码回复"} ("元素"), timeout in ms (-1)=10 ("超时毫秒(-1)")) -> ()  [unwired: 1 in, 3 out]
              }
            }
          }
          frame "读二维码" {
            w6624 = u16 0 items=["byte", "word", "Dword"] ("数据类型")
            w6620 = u8 132 items=["I/O (P)"=128, "Input (I)"=129, "Output (Q)"=130, "Bit Memory (M)"=131, "Data (DB)"=132, "Instance Data (DI)"=133, "Local Data (L)"=134, "Predecessor Local Data (VL)"=135] ("寄存器类型")
            n1235 = call "S7_Read.vi"("TCP"=w6619, "DB #"=u16 20, "读取长度"=u16 17, "寄存器类型"=w6620, "起始地址"=u32 24, "数据类型"=w6624) -> ("TCP"=w6618:refnum<k5>, "数据"=w6625:u32[], "error out"=w6627:errorcluster)  [unwired: 6 in, 1 out]
            n1236 = To Unsigned Word Integer(number=w6625) -> (unsigned 16bit integer=w6626:u16[])
            n1237 = call "还原为字符串.vi"("error in (no error)"=w6627, "输入数组"=w6626) -> ("error out"=w6611:errorcluster, "字符串"=w6612:string)  [unwired: 8 in]
            n1238 = Match Pattern(string=w6612, regular expression=" " ("正则表达式")) -> (before substring=w6609:string)  [unwired: 1 in, 3 out]
            n1239 = flat-sequence {
              tunnel: w6611 -> [w6629]
              tunnel: [w6629] -> w6610
              tunnel: w6609 -> [w6628]
              tunnel: [w6632] -> w6615
              tunnel: w6610 -> [w6630]
              frame #0 {
                "201二维码" <- w6628
              }
              frame #1 {
                n1240 = property on="ST201扫码请求(事件)" class="Bool (严格)"(error in=w6630, "Val(Sgnl)"=TRUE ("值(信号)")) -> (error out=w6632:errorcluster)  [unwired: 1 in, 1 out]
              }
            }
          }
          frame "扫码回复" {
            n1241 = Array Size(array=w6635) -> (size(s)=w6636:i32)
            n1242 = case shown="3, 默认" w6636 {
              tunnel: w6635 -> [w6643 w6677]
              tunnel: w6639 -> [w6644 w6664]
              tunnel: [w6646 w6655] -> w6638
              tunnel: [w6645 w6654] -> w6637
              tunnel: [w6642 w6653] -> w6633
              frame 1 {
                w6649 = u8 132 items=["I/O (P)"=128, "Input (I)"=129, "Output (Q)"=130, "Bit Memory (M)"=131, "Data (DB)"=132, "Instance Data (DI)"=133, "Local Data (L)"=134, "Predecessor Local Data (VL)"=135] ("寄存器类型")
                w6648 = u16 1 items=["byte", "word", "Dword"] ("数据类型")
                n1243 = Index Array(array=w6643) -> (element=w6642:string)  [unwired: 1 in]
                n1244 = Decimal String To Number(string=w6642, default (0L)=u32 0 ("默认(0 I32)")) -> (number=w6652:u32)  [unwired: 1 in, 1 out]
                n1245 = call "S7_Write.vi"("TCP"=w6644, "寄存器类型"=w6649, "DB #"=u16 20, "写入地址"=u32 2, "数据类型"=w6648, "写入数据"=w6652) -> ("TCP"=w6646:refnum<k5>, "error out"=w6645:errorcluster)  [unwired: 7 in, 1 out]
              }
              frame 3, Default {
                w6667 = u8 132 items=["I/O (P)"=128, "Input (I)"=129, "Output (Q)"=130, "Bit Memory (M)"=131, "Data (DB)"=132, "Instance Data (DI)"=133, "Local Data (L)"=134, "Predecessor Local Data (VL)"=135] ("寄存器类型")
                w6666 = u16 1 items=["byte", "word", "Dword"] ("数据类型")
                w6674 = u8 132 items=["I/O (P)"=128, "Input (I)"=129, "Output (Q)"=130, "Bit Memory (M)"=131, "Data (DB)"=132, "Instance Data (DI)"=133, "Local Data (L)"=134, "Predecessor Local Data (VL)"=135] ("寄存器类型")
                w6675 = u16 1 items=["byte", "word", "Dword"] ("数据类型")
                w6681 = u8 132 items=["I/O (P)"=128, "Input (I)"=129, "Output (Q)"=130, "Bit Memory (M)"=131, "Data (DB)"=132, "Instance Data (DI)"=133, "Local Data (L)"=134, "Predecessor Local Data (VL)"=135] ("寄存器类型")
                w6680 = u16 1 items=["byte", "word", "Dword"] ("数据类型")
                n1246 = Index Array(array=w6677) -> (element #1=w6653:string, element #2=w6660:string, element #3=w6659:string)  [unwired: 3 in]
                n1247 = Equal?(x=w6659, y="OK") -> (x = y?=w6657:bool)
                n1248 = Decimal String To Number(string=w6660, default (0L)=u32 0 ("默认(0 I32)")) -> (number=w6661:u32)  [unwired: 1 in, 1 out]
                n1249 = case shown="假" w6657 {
                  tunnel: [u32 2 ("写入数据") u32 1 ("写入数据")] -> w6656
                  frame False {
                  }
                  frame True {
                  }
                }
                n1250 = call "S7_Write.vi"("TCP"=w6664, "寄存器类型"=w6681, "DB #"=u16 20, "写入地址"=u32 8, "数据类型"=w6680, "写入数据"=w6661) -> ("TCP"=w6671:refnum<k5>, "error out"=w6672:errorcluster)  [unwired: 7 in, 1 out]
                n1251 = call "S7_Write.vi"("TCP"=w6671, "寄存器类型"=w6674, "DB #"=u16 20, "写入地址"=u32 10, "数据类型"=w6675, "写入数据"=w6656, "error in"=w6672) -> ("TCP"=w6663:refnum<k5>, "error out"=w6662:errorcluster)  [unwired: 6 in, 1 out]
                n1252 = Decimal String To Number(string=w6653, default (0L)=u32 0 ("默认(0 I32)")) -> (number=w6670:u32)  [unwired: 1 in, 1 out]
                n1253 = call "S7_Write.vi"("TCP"=w6663, "寄存器类型"=w6667, "DB #"=u16 20, "写入地址"=u32 2, "数据类型"=w6666, "写入数据"=w6670, "error in"=w6662) -> ("TCP"=w6655:refnum<k5>, "error out"=w6654:errorcluster)  [unwired: 6 in, 1 out]
              }
            }
            "扫码请求回复201" <- w6633
            n1254 = Bundle By Name(cluster=w6634, "扫码超时1"=w6633) -> ()  [unwired: 1 out]
          }
          frame "-------------" {
          }
          frame "读数据保存请求" {
            w6718 = u16 0 items=["byte", "word", "Dword"] ("数据类型")
            w6720 = u8 132 items=["I/O (P)"=128, "Input (I)"=129, "Output (Q)"=130, "Bit Memory (M)"=131, "Data (DB)"=132, "Instance Data (DI)"=133, "Local Data (L)"=134, "Predecessor Local Data (VL)"=135] ("寄存器类型")
            n1255 = call "S7_Read.vi"("TCP"=w6710, "DB #"=u16 20, "读取长度"=u16 1, "寄存器类型"=w6720, "起始地址"=u32 0, "数据类型"=w6718) -> ("TCP"=w6709:refnum<k5>, "数据"=w6715:u32[], "error out"=w6708:errorcluster)  [unwired: 6 in, 1 out]
            n1256 = Index Array(array=w6715, index=0 ("索引")) -> (element=w6713:u32)
            n1257 = Number To Boolean Array(number=w6713) -> (Boolean array=w6712:bool[])
            n1258 = Unbundle By Name(w6691) -> ("数据保存超时1"=w6692:string)
            n1259 = Index Array(array=w6712, index=1 ("索引")) -> (element=w6697:bool)
            "ST201数据读取" <- w6697
            n1260 = Not Equal?(x=w6692, y="999") -> (x != y?=w6694:bool)
            n1261 = Not(x=w6694) -> (.not. x?=w6695:bool)
